vi "GetCtrlRefFromWaitOccurance.vi"(0 "VI Path To Open":path=path "D:/Work/Tests/3.0/FlexLVAdapter/Refnums/OccuranceRefnum/WaitOccurance.vi") -> (1 "VI Refnum":refnum<vi>, 2 "String Output Refnum":refnum<vi>, 3 "error out":errorcluster)   [LabVIEW 2010]
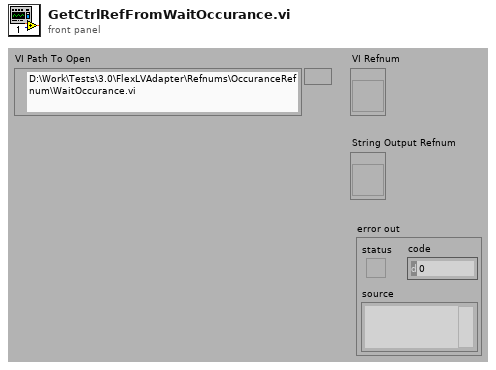
[diagram p1: front panel]
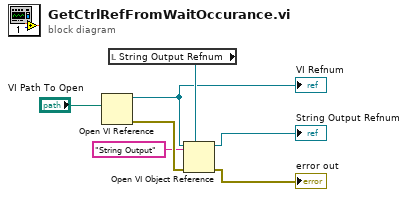
[diagram p0: block diagram]
diagram:
  n1 = Open VI Reference(vi path="VI Path To Open") -> (vi reference=w1:refnum<vi>, error out=w6:errorcluster)  [unwired: 2 in, 3 out]
  "VI Refnum" <- w1
  n2 = local read "String Output Refnum"() -> (w2:refnum<vi>)
  n3 = Open VI Object Reference(7:w2, 8:w6, 10:"String Output" ("name/order"), 11:w1) -> (0:→"error out":errorcluster, 3:→"String Output Refnum":refnum<vi>)
